vi "UsrProfiles-Paste profile.vi"   [LabVIEW 2013]
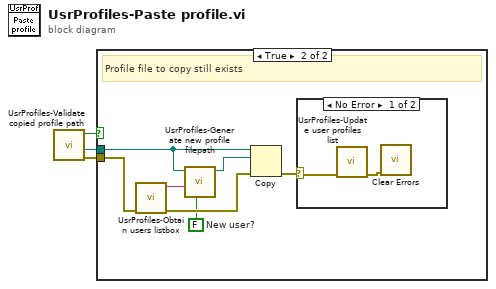
[diagram p0: block diagram]
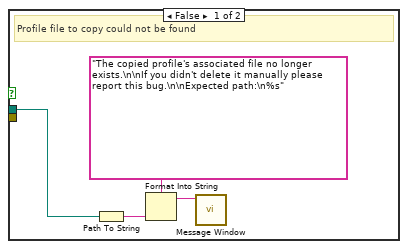
[diagram p2: hidden frame]
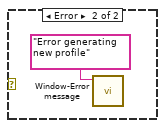
[diagram p3: hidden frame]
diagram:
  n1 = call "UsrProfiles-Validate copied profile path.vi"() -> ("error out"=w2:errorcluster, "Copied profile file path"=w3:path, "copied profile file still exists"=w1:bool)  [unwired: 9 in]
  n2 = case shown="True" w1 {
    tunnel: w3 -> [w5 w13]
    tunnel: w2 -> [_ w11]
    frame False {
      # "Profile file to copy could not be found"
      n3 = Path To String(path=w5) -> (string=w7:string)
      n4 = Format Into String(format string="The copied profile's associated file no longer exists.\n\nIf you didn't delete it manually please report this bug.\n\nExpected path:\n%s", w7) -> (resulting string=w6:string)  [unwired: 2 in, 1 out]
      n5 = call "Message Window.vi"("Message string"=w6) -> ()  [unwired: 10 in, 1 out]
    }
    frame True {
      w8 = FALSE  # New user?
      # "Profile file to copy still exists"
      n6 = call "UsrProfiles-Obtain users listbox.vi"("error in (no error)"=w11) -> ("error out"=w10:errorcluster, "Selected user's name"=w14:string)  [unwired: 7 in, 2 out]
      n7 = call "UsrProfiles-Generate new profile filepath.vi"("New user"=w8, "Destination User name"=w14, "Copied profile's filepath"=w13) -> ("Filepath of profile to be created"=w12:path)  [unwired: 8 in]
      n8 = Copy(8:w10, 10:w12, 11:w13) -> (0:w9:errorcluster)  [unwired: 2 in, 2 out]
      n9 = case shown="No Error" w9 {
        selector: w9 -> [w16 _]
        frame No Error {
          n10 = call "UsrProfiles-Update user profiles list.vi"("error in"=w16) -> ("error out"=w15:errorcluster)  [unwired: 10 in]
          n11 = call <vilib>:"Clear Errors.vi"("error in (no error)"=w15) -> ()  [unwired: 6 in, 1 out]
        }
        frame Error {
          n12 = call "Window-Error message.vi"("Message"="Error generating new profile") -> ()  [unwired: 10 in, 1 out]
        }
      }
    }
  }
